vi "get command from counter cluster.vi"(6 "tracking?":bool, 7 "counting photons?":bool, 10 "counter cluster":T2) -> (2 "command":T1)   [LabVIEW 2010]
uses:
  counter_cluster_tagResonant.ctl
  scan message.ctl
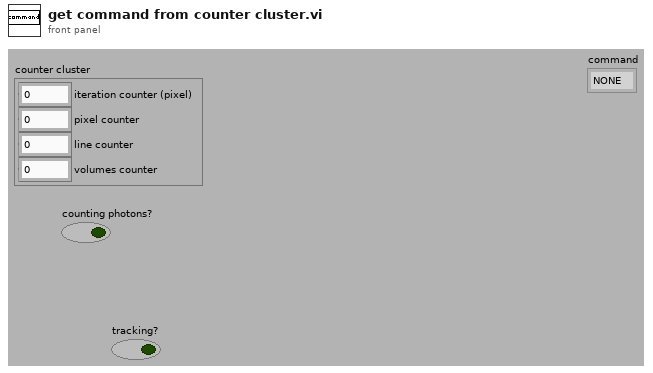
[diagram p1: front panel]
types:
  T1 = typedef "scan message.ctl" = enum8{"NONE", "VOLUME START", "LINE START", "LINE START TRACKING", "XKALMAN", "YKALMAN", "ZKALMAN"}
  T2 = typedef "counter_cluster_tagResonant.ctl" = cluster{"iteration counter (pixel)":u16, "pixel counter":u16, "line counter":i16, "volumes counter":u16}
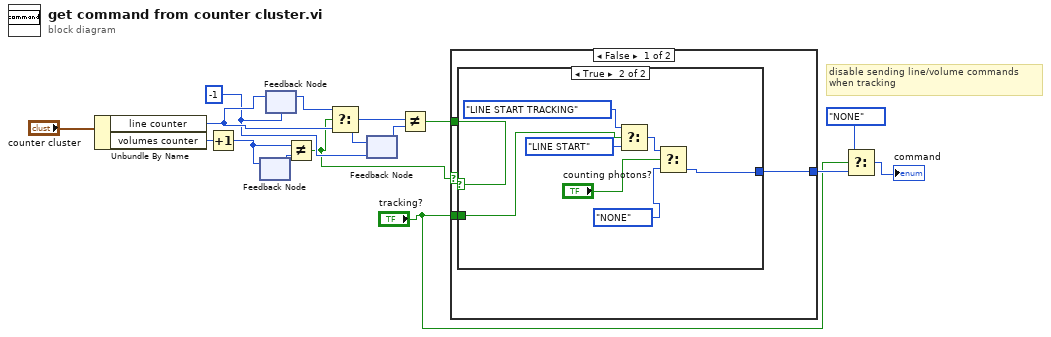
[diagram p0: block diagram]
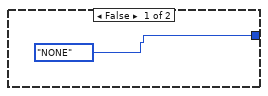
[diagram p2: hidden frame]
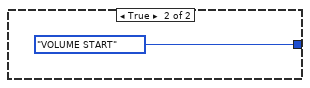
[diagram p3: hidden frame]
diagram:
  w7 = i16 -1 ("line counter")
  # "disable sending line/volume commands\nwhen tracking"
  n1 = Unbundle By Name("counter cluster") -> ("line counter"=w11:i16, "volumes counter"=w13:u16)
  n2 = Increment(x=w13) -> (x+1=w4:u16)
  n3 = feedback #1() -> (w12:u16)  [unwired: 1 in]
  n4 = feedback-in #1(w4) -> ()
  n5 = feedback #2(w7) -> (w10:i16)
  n6 = feedback-in #2(w11) -> ()
  n7 = Not Equal?(x=w4, y=w12) -> (x != y?=w6:bool)
  n8 = Select(t=w10, s=w6, f=w11) -> (s? t:f=w8:i16)
  n9 = feedback #3(w7) -> (w9:i16)
  n10 = feedback-in #3(w8) -> ()
  n11 = Not Equal?(x=w8, y=w9) -> (x != y?=w5:bool)
  n12 = case shown="False" w6 {
    tunnel: [w17 scan_message."VOLUME START" ("Enum")] -> w14
    tunnel: w5 -> [w18 _]
    tunnel: "tracking?" -> [w16 _]
    frame False {
      n13 = case shown="True" w18 {
        tunnel: [scan_message."NONE" ("f") w26] -> w17
        tunnel: w16 -> [_ w20]
        frame False {
        }
        frame True {
          n14 = Select(t=scan_message."LINE START TRACKING" ("Enum"), s=w20, f=scan_message."LINE START" ("Enum")) -> (s? t:f=w21:T1)
          n15 = Select(t=w21, s="counting photons?", f=scan_message."NONE") -> (s? t:f=w26:T1)
        }
      }
    }
    frame True {
    }
  }
  n16 = Select(t=scan_message."NONE", s="tracking?", f=w14) -> (s? t:f=→"command":T1)
